vi "CTR_8254ModeLoad.vi"(7 "DeviceIndex":u32, 8 "error in (no error)":errorcluster) -> (0 "error out":errorcluster, 2 "Actual WriteClockHz":dbl, 3 "Actual ReadClockHz":dbl)   [LabVIEW 2012]
doc: "unsigned long CTR_8254ModeLoad(\nunsigned long DeviceIndex - number from 0-31 indicating on which device you wish to mode\nand load an 8254 counter\nunsigned long BlockIndex - number indicating which 8254 you wish to mode and load\nunsigned long CounterIndex - number from 0-2 indicating which counter on the specified 8254\nyou wish to mode and load\n18\nunsigned long Mode - a number from 0-5 specifying which 8254 mode you want the specified\ncounter to be\nunsigned short LoadValue - a number from 0 to 65535 which you wish loaded into the specified\ncounter\n)"
uses:
  Controls/Counter Modes.ctl
  Windows/System32/AIOUSB.dll
panel:
  in  "LoadValue":u32
  in  "Mode":T1
  in  "CounterIndex":u32
  in  "BlockIndex":u32
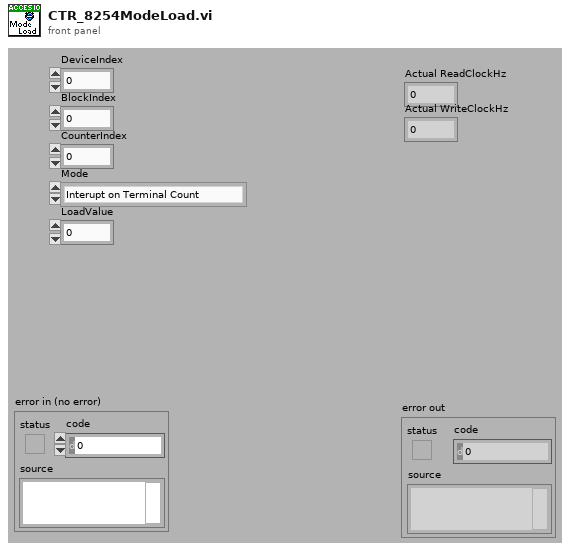
[diagram p1: front panel]
types:
  T1 = typedef "Counter Modes.ctl" = enum16{"Interupt on Terminal Count", "Hardware Retriggerable, One-shot", "Rate Generator", "Squre Wave", "Software Triggered", "Hardware Triggered"}
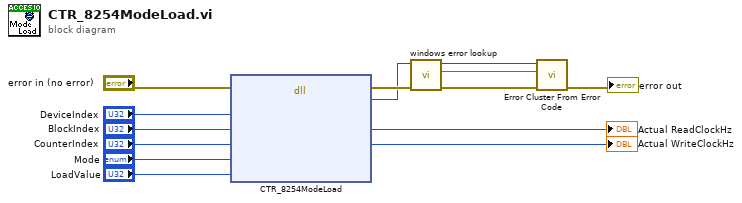
[diagram p0: block diagram]
diagram:
  n1 = dll-call lib="C:/Windows/System32/AIOUSB.dll" fn="CTR_8254ModeLoad"(error in="error in (no error)", "DeviceIndex"="DeviceIndex", "BlockIndex"="BlockIndex", "CounterIndex"="CounterIndex", "Mode"="Mode", "LoadValue"="LoadValue") -> (error out=w10:errorcluster, "return type"=w9:u32, "BlockIndex"=→"Actual ReadClockHz":u32, "CounterIndex"=→"Actual WriteClockHz":u32)  [unwired: 5 in, 1 out]
  n2 = call "windows error lookup.vi"("error in (no error)"=w10, "Error Code"=w9) -> ("error out"=w12:errorcluster, "error message (\"\")"=w13:string)  [unwired: 8 in]
  n3 = call <vilib>:"Error Cluster From Error Code.vi"("error in (no error)"=w12, "error message (\"\")"=w13, "error code (0)"=w9) -> ("error out"=→"error out":errorcluster)  [unwired: 6 in]
